vi "FilterConnections.vi"(1 "Selected Connections":string[](array[string])) -> (0 "Filtered Connections":string[](array[string]))   [LabVIEW 2015]
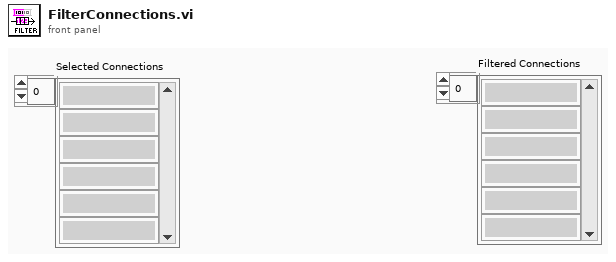
[diagram p1: front panel]
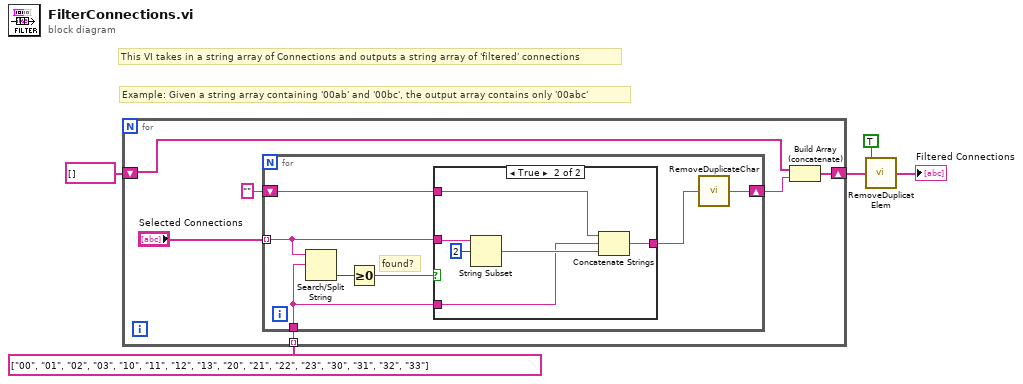
[diagram p0: block diagram]
diagram:
  # "Example: Given a string array containing '00ab' and '00bc', the output array contains only '00abc'"
  # "This VI takes in a string array of Connections and outputs a string array of 'filtered' connections"
  n1 = for {
    tunnel: string[] ["00", "01", "02", "03", "10", "11", "12", "13", "20", "21", "22", "23", "30", "31", "32", "33"] -> [w10] mode=indexing
    shift-right: [w7] -> w3
    shift-left: string[] [] -> [w6]
    n2 = for {
      tunnel: "Selected Connections" -> [w16] mode=indexing
      tunnel: w10 -> [w15]
      shift-right: [w12] -> w8
      shift-left: "" -> [w14]
      # "found?"
      n3 = Search/Split String(string=w16, search string/char (-)=w15) -> (offset of match=w18:i32)  [unwired: 1 in, 2 out]
      n4 = Greater Or Equal To 0?(x=w18) -> (x >= 0?=w17:bool)
      n5 = case shown="True" w17 {
        tunnel: w16 -> [_ w24]
        tunnel: w15 -> [_ w22]
        tunnel: [w19 w21] -> w13
        tunnel: w14 -> [w19 w20]
        frame False {
        }
        frame True {
          n6 = String Subset(string=w24, offset (0)=2) -> (substring=w23:string)  [unwired: 1 in]
          n7 = Concatenate Strings(w20, w22, w23) -> (w21:string)
        }
      }
      n8 = call "RemoveDuplicateChar.vi"("Input String"=w13) -> ("Discrete String"=w12:string)
    }
    n9 = Build Array (concatenate)(w6, w8) -> (w7:string[])
  }
  n10 = call "RemoveDuplicatElem.vi"("Input Array"=w3, "Remove Empty Strings?"=TRUE) -> ("Discrete Array"=→"Filtered Connections":string[])
